vi "MatrixMultiblock.vi"(7 "Induction Matrix Build Properties":T1) -> ()   [LabVIEW 2024]
uses:
  Induction Matrix Build Properties.ctl
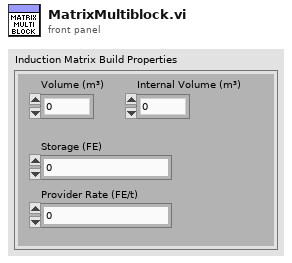
[diagram p1: front panel]
types:
  T1 = typedef "Induction Matrix Build Properties.ctl" = cluster{"Internal Volume (m³)":i32, "Volume (m³)":i32, "Storage (FE)":ext, "Provider Rate (FE/t)":ext}
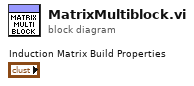
[diagram p0: block diagram]
diagram:
